vi "P5.vi"() -> ()   [LabVIEW 2019]
panel:
  in  "E Button":bool
  in  "D Button":bool
  in  "C Button":bool
  in  "B Button":bool
  in  "Exit Button":bool
  out "String":string
  in  "A Button":bool
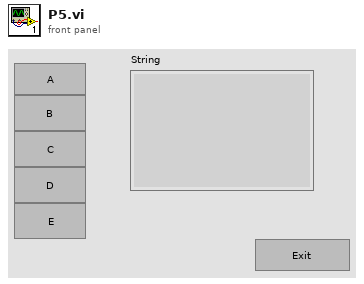
[diagram p1: front panel]
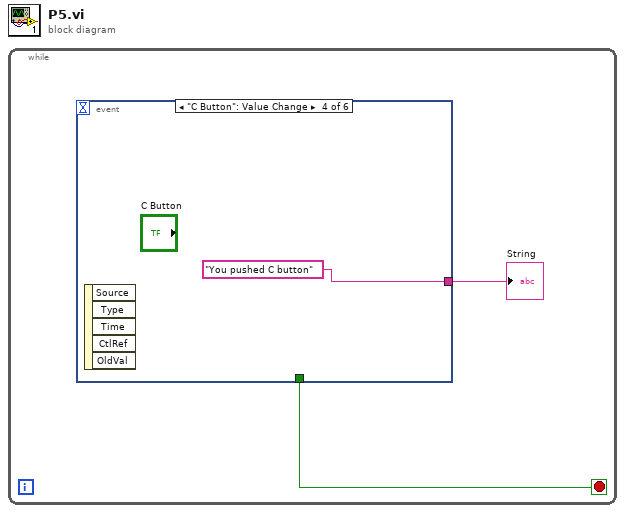
[diagram p0: block diagram]
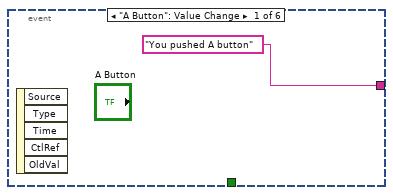
[diagram p2: hidden frame]
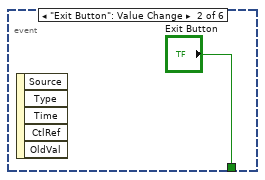
[diagram p3: hidden frame]
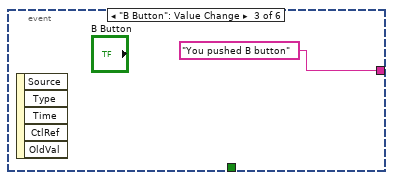
[diagram p4: hidden frame]
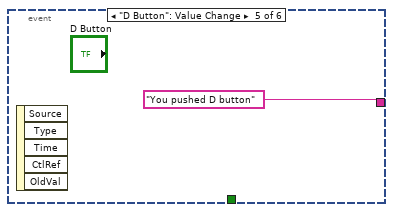
[diagram p5: hidden frame]
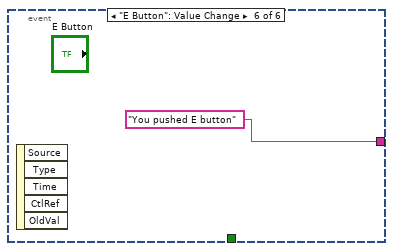
[diagram p6: hidden frame]
diagram:
  n1 = while {
    stop <- w2 stop-if-true
    n2 = event shown="[3] \"C Button\": Value Change" {
      selector: _ -> [_ _ _ _ _ _]
      dyn-events: _ -> [_ _ _ _ _ _]
      timeout: _ -> [_ _ _ _ _ _]
      tunnel: [_ "Exit Button" _ _ _ _] -> w2
      tunnel: ["You pushed A button" ("String") _ "You pushed B button" "You pushed C button" "You pushed D button" "You pushed E button"] -> w1
      event "A Button": Value Change {
        n3 = event-data() -> ()  [unwired: 1 in, 5 out]
      }
      event "Exit Button": Value Change {
        n4 = event-data() -> ()  [unwired: 1 in, 5 out]
      }
      event "B Button": Value Change {
        n5 = event-data() -> ()  [unwired: 1 in, 5 out]
      }
      event "C Button": Value Change {
        n6 = event-data() -> ()  [unwired: 1 in, 5 out]
      }
      event "D Button": Value Change {
        n7 = event-data() -> ()  [unwired: 1 in, 5 out]
      }
      event "E Button": Value Change {
        n8 = event-data() -> ()  [unwired: 1 in, 5 out]
      }
    }
    "String" <- w1
  }
